vi "loadDataNodeBegin.vi"(8 "error in (no error)":errorcluster, 10 "XML Refnum in":refnum<file>, 11 "Categories in":refnum<class "Categories.lvclass">) -> (0 "error out":errorcluster, 2 "XML Refnum out":refnum<file>, 3 "Categories out":refnum<class "Categories.lvclass">)   [LabVIEW 2013, in "Categories.lvclass"]
doc: "Part of the file loading process. Occurs at the beginning of a node being loaded. Loads the common xceDataNode data name and description."
uses:
  Categories.lvclass
  Categories.lvclass/Categories.ctl
  xCE/xceNode/xceNode.lvclass
  XML Parser/XML Parser.lvclass
panel:
  out "Token Found":bool
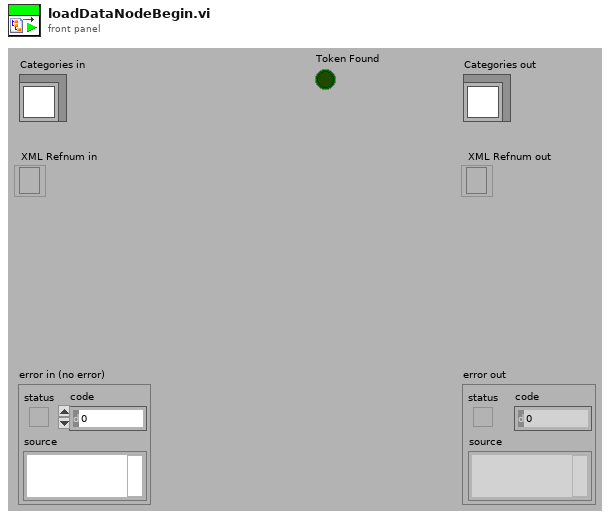
[diagram p1: front panel]
types:
  T1 = typedef "enum_Symbols.ctl" = enum16{"Default", "Analog Input", "Analog Output", "Digital Input", "Digital Output", "PWM Input", "PWM Output"}
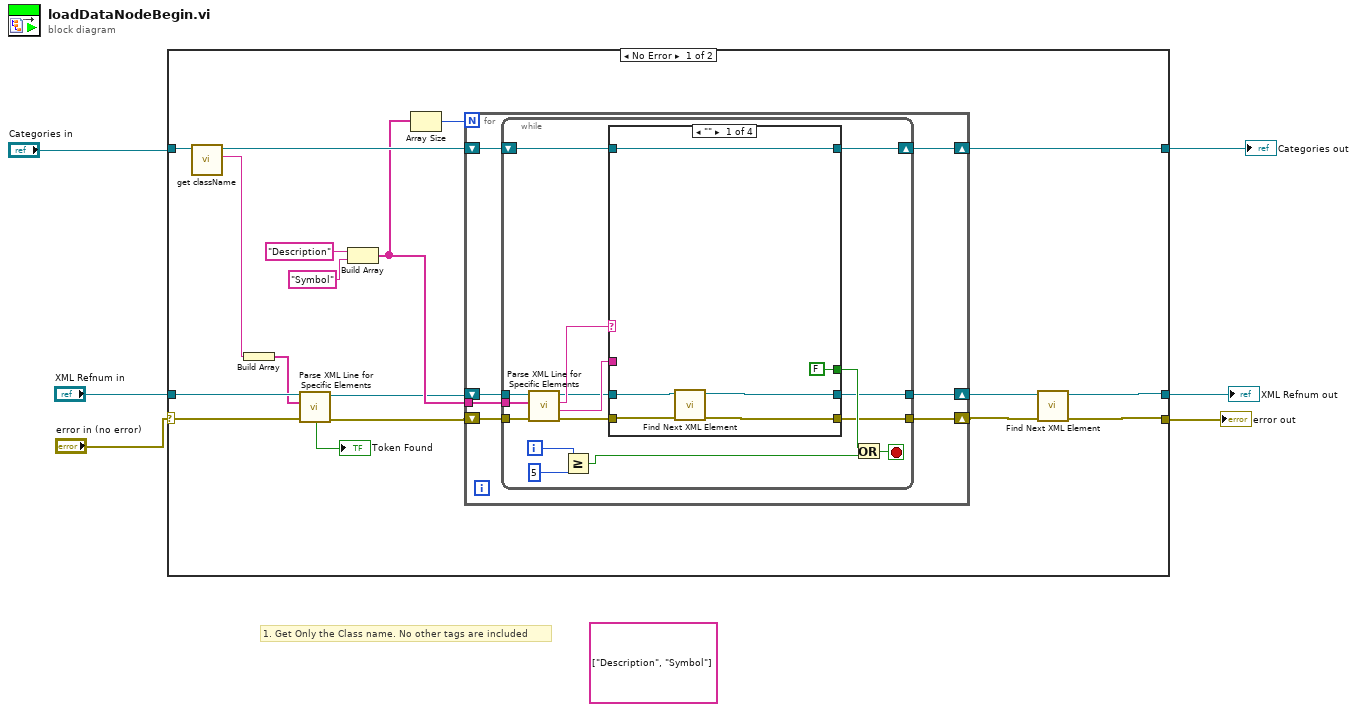
[diagram p0: block diagram]
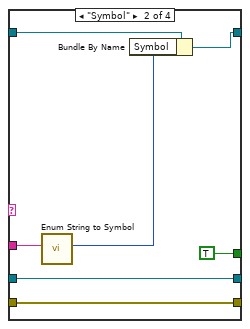
[diagram p2: hidden frame]
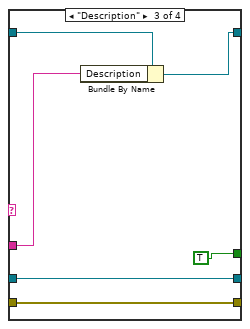
[diagram p3: hidden frame]
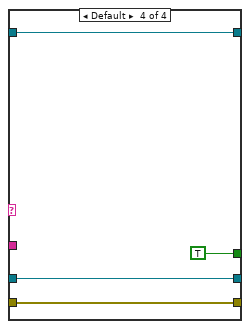
[diagram p4: hidden frame]
diagram:
  (unwired) string[] ["Description", "Symbol"] ("Token List")
  # "1. Get Only the Class name. No other tags are included"
  n1 = case shown="No Error" "error in (no error)" {
    selector: "error in (no error)" -> [w16 w73]
    tunnel: [w8 w73] -> w3
    tunnel: [w22 w72] -> w1
    tunnel: "Categories in" -> [w24 w72]
    tunnel: "XML Refnum in" -> [w17 w71]
    tunnel: [w7 w71] -> w2
    frame No Error {
      n2 = call "get className.vi"("xceNode in"=w24) -> ("Class name"=w15:string, "xceNode out"=w23:refnum<class "Categories.lvclass">)  [unwired: 8 in, 1 out]
      n3 = Build Array(w15) -> (w14:string[])
      n4 = call "Parse XML Line for Specific Elements.vi"("error in (no error)"=w16, "Elements"=w14, "XML Refnum in"=w17) -> ("error out"=w13:errorcluster, "XML Refnum out"=w12:refnum<file>, "Element Found"=→"Token Found":bool)  [unwired: 4 in, 2 out]
      n5 = Build Array("Description" ("regular expression"), "Symbol" ("regular expression")) -> (w19:string[])
      n6 = Array Size(array=w19) -> (size(s)=w18:i32)
      n7 = for {
        N: w18 -> [_]
        tunnel: w19 -> [w31]
        shift-right: [w26] -> w22
        shift-left: w23 -> [w28]
        shift-right: [w27] -> w10
        shift-left: w12 -> [w30]
        shift-right: [w25] -> w9
        shift-left: w13 -> [w29]
        n8 = while {
          tunnel: w31 -> [w47]
          tunnel: w30 -> [w46]
          tunnel: w29 -> [w45]
          shift-right: [w40] -> w26
          shift-left: w28 -> [w42]
          tunnel: [w32] -> w27
          tunnel: [w33] -> w25
          i -> [w44]
          stop <- w37 stop-if-true
          n9 = call "Parse XML Line for Specific Elements.vi"("error in (no error)"=w45, "Elements"=w47, "XML Refnum in"=w46) -> ("error out"=w34:errorcluster, "Value"=w36:string, "Element Name"=w41:string, "XML Refnum out"=w35:refnum<file>)  [unwired: 4 in, 1 out]
          n10 = Greater Or Equal?(x=w44, y=5) -> (x >= y?=w38:bool)
          n11 = case shown="\"\"" w41 {
            tunnel: w42 -> [w53 w60 w66 w70]
            tunnel: [w53 w59 w65 w70] -> w40
            tunnel: [FALSE TRUE TRUE TRUE] -> w39
            tunnel: w36 -> [_ w55 w64 _]
            tunnel: w35 -> [w51 w57 w62 w68]
            tunnel: w34 -> [w50 w56 w61 w67]
            tunnel: [w48 w56 w61 w67] -> w33
            tunnel: [w49 w57 w62 w68] -> w32
            frame "" {
              n12 = call "Find Next XML Element.vi"("error in (no error)"=w50, "XML Fine In"=w51) -> ("error out"=w48:errorcluster, "XML Fine Out"=w49:refnum<file>)  [unwired: 7 in, 1 out]
            }
            frame "Symbol" {
              n13 = call "Enum String to Symbol.vi"("Symbol String In"=w55) -> ("Symbol Enum Out"=w54:T1)  [unwired: 10 in]
              n14 = Bundle By Name(cluster=w60, "Symbol"=w54) -> (w59:refnum<class "Categories.lvclass">)
            }
            frame "Description" {
              n15 = Bundle By Name(cluster=w66, "Description"=w64) -> (w65:refnum<class "Categories.lvclass">)
            }
            frame Default {
            }
          }
          n16 = Or(x=w39, y=w38) -> (x .or. y?=w37:bool)
        }
      }
      n17 = call "Find Next XML Element.vi"("error in (no error)"=w9, "XML Fine In"=w10) -> ("error out"=w8:errorcluster, "XML Fine Out"=w7:refnum<file>)  [unwired: 7 in, 1 out]
    }
    frame Error {
    }
  }
  "error out" <- w3
  "Categories out" <- w1
  "XML Refnum out" <- w2
